vi "Less Than.vi"(1 "compare b":string, 2 "compare a":string, 3 "AoC22.lvlib:Packet Compare.lvclass":refnum<class "Packet Compare.lvclass">) -> (0 "A < B?":bool)   [LabVIEW 2022 SP3, in "AoC22.lvlib" / "Packet Compare.lvclass"]
uses:
  Packet Compare.lvclass
  Packet Compare.lvclass/Packet Compare.ctl
  AoC22.lvlib
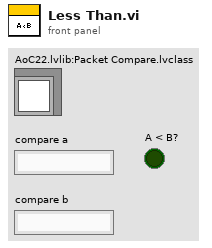
[diagram p1: front panel]
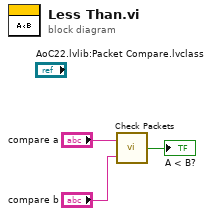
[diagram p0: block diagram]
diagram:
  n1 = call "Check Packets.vi"("A"="compare b", "B"="compare a") -> ("A < B?"=→"A < B?":bool)
